vi "FXP Test.vi"() -> ()   [LabVIEW 2020]
uses:
  <vilib>/rvi/eio/common/nirviEmuTemplateMethod_errors.vi
  <vilib>/eio/EIONode/EIONode.xnode
panel:
  in  "Mod2/AO0":fxp<+,20,-5> format="%.24g"
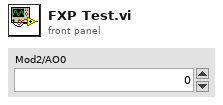
[diagram p1: front panel]
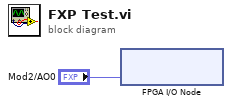
[diagram p0: block diagram]
diagram:
  n1 = xnode "FPGA I/O Node"("Mod2/AO0"="Mod2/AO0") -> ()  [unwired: 1 in, 1 out]
